vi "onDependencyConfigChanged.vi"(4 "Source GUID":string, 6 "keys changed":string[](array[string]), 7 "Propagate to caller? (T)":bool=TRUE, 8 "error in":errorcluster, 9 "Dependency":refnum<class "SMO.lvclass">, 11 "SMO in":refnum<class "SMO.lvclass">) -> (0 "error out":errorcluster, 3 "SMO out":refnum<class "SMO.lvclass">)   [LabVIEW 2013, in "SMO.lvclass"]
uses:
  SMO.lvclass
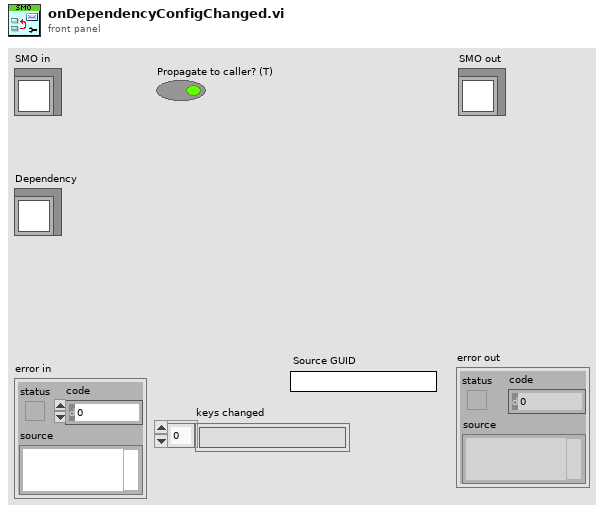
[diagram p1: front panel]
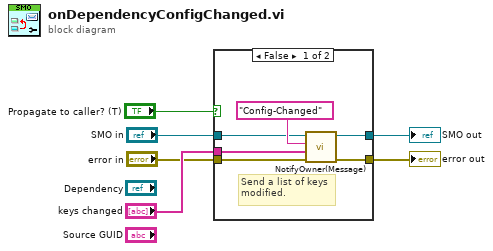
[diagram p0: block diagram]
diagram:
  n1 = case shown="False" "Propagate to caller? (T)" {
    tunnel: "SMO in" -> [w11 w14]
    tunnel: [w10 w14] -> w3
    tunnel: "error in" -> [w9 w13]
    tunnel: [w8 w13] -> w1
    tunnel: "keys changed" -> [w7 _]
    frame False {
      # "Send a list of keys\nmodified."
      n2 = call "NotifyOwner(Message).vi"("error in (no error)"=w9, "Payload"=w7, "Message (empty : payload label)"="Config-Changed", "SMO in"=w11) -> ("error out"=w8:errorcluster, "SMO out"=w10:refnum<class "SMO.lvclass">)  [unwired: 6 in]
    }
    frame True {
      # "No notification change\nevent to caller on\nprivate config change"
    }
  }
  "SMO out" <- w3
  "error out" <- w1
